vi "Get Cell Q.vi"(8 "error in":errorcluster, 11 "PAS Data in":refnum<class "PAS Data.lvclass">) -> (0 "error out":errorcluster, 2 "Q":sgl, 3 "PAS Data out":refnum<class "PAS Data.lvclass">)   [LabVIEW 2014, in "PAS Library.lvlib" / "PAS Data.lvclass"]
uses:
  PAS Data.lvclass
  PAS Data.lvclass/PAS Data.ctl
  Cell/PAS Cell Data.lvclass
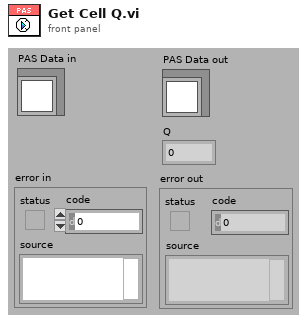
[diagram p1: front panel]
types:
  T1 = cluster{"f0":sgl, "IA":sgl, "Q":sgl, "max":dbl[], "noiseLim":dbl, "ext":dbl}
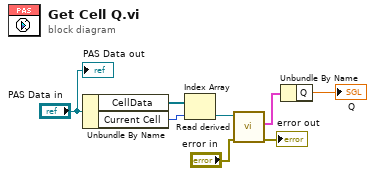
[diagram p0: block diagram]
diagram:
  n1 = Unbundle By Name("PAS Data in") -> ("CellData"=w7:refnum<class "PAS Cell Data.lvclass">[], "Current Cell"=w6:i32)
  n2 = Index Array(array=w7, index=w6) -> (element=w5:refnum<class "PAS Cell Data.lvclass">)
  n3 = call "Read derived.vi"("error in"="error in", "PAS Cell Data in"=w5) -> ("error out"=→"error out":errorcluster, "derived"=w2:T1)  [unwired: 7 in, 1 out]
  n4 = Unbundle By Name(w2) -> ("Q"=→"Q":sgl)
  "PAS Data out" <- "PAS Data in"
